vi "setCamRamSegment.vi"(0 "Camera in":refnum<class "Camera.lvclass">, 5 "segment":u16=1, 11 "error in (no error)":errorcluster) -> (4 "Camera out":refnum<class "Camera.lvclass">, 15 "error out":errorcluster)   [LabVIEW 2019, in "Camera.lvclass"]
doc: "Sets the number of the current CAMRAM segment. Subsequent recordings will use this segment, and images will be read from this segment. For cameras with internal memory only."
uses:
  Camera.lvclass
  Camera.lvclass/Camera.ctl
  pco.sdk/StorageControl/StorageControl.lvlib
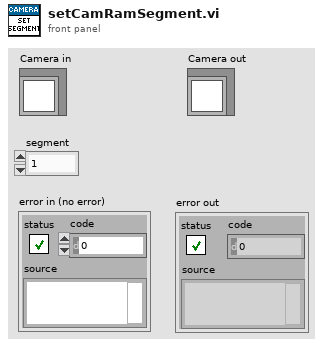
[diagram p1: front panel]
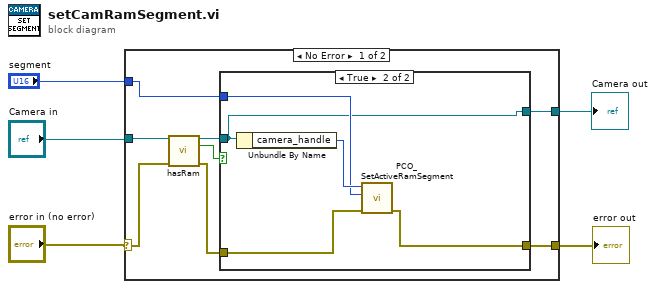
[diagram p0: block diagram]
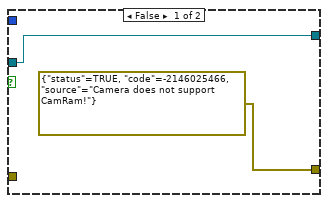
[diagram p2: hidden frame]
diagram:
  n1 = case shown="No Error" "error in (no error)" {
    selector: "error in (no error)" -> [w12 w22]
    tunnel: [w7 w22] -> w3
    tunnel: [w6 w21] -> w4
    tunnel: "Camera in" -> [w13 w21]
    tunnel: "segment" -> [w8 _]
    frame No Error {
      n2 = call-dynamic "hasRam.vi"("Camera in"=w13, "error in (no error)"=w12) -> ("Camera out"=w9:refnum<class "Camera.lvclass">, "hasRam"=w10:bool, "error out"=w11:errorcluster)  [unwired: 11 in]
      n3 = case shown="True" w10 {
        tunnel: w11 -> [_ w20]
        tunnel: w9 -> [w14 w16]
        tunnel: w8 -> [_ w17]
        tunnel: [errorcluster {"status"=TRUE, "code"=-2146025466, "source"="Camera does not support CamRam!"} ("error constant") w19] -> w7
        tunnel: [w14 w16] -> w6
        frame False {
        }
        frame True {
          n4 = Unbundle By Name(w16) -> ("camera_handle"=w18:u64)
          n5 = call "PCO_SetActiveRamSegment.vi"("error in (no error)"=w20, "wActSeg"=w17, "ph"=w18) -> ("error out"=w19:errorcluster)  [unwired: 6 in, 2 out]
        }
      }
    }
    frame Error {
    }
  }
  "error out" <- w3
  "Camera out" <- w4
